vi "Match-Value Image (Colour).vi"(8 "error in (no error)":errorcluster, 9 "Value":u32(colorbox), 10 "Match":T1, 11 "ARGB Image Source":T2) -> (0 "error out":errorcluster, 3 "Match Destination (duplicate)":T1)   [LabVIEW 2020, in "g_ar_toolkit.image.lvlib"]
uses:
  g_ar_toolkit.image.lvlib
  ARGB Image.ctl
  Greyscale Image.ctl
  5701baee-35e2-4306-9a77-a9fdbb5b3a7f.vi
  g_ar_toolkit.common/Module Path.vi
  <vilib>/Utility/error.llb/Error Cluster From Error Code.vi
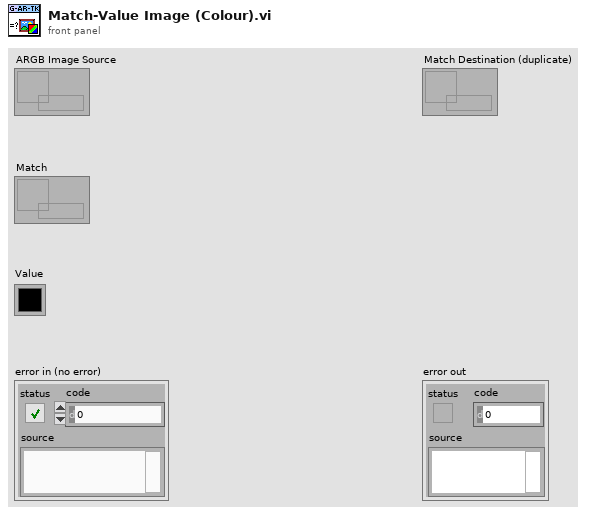
[diagram p1: front panel]
types:
  T1 = typedef "g_ar_toolkit.image.lvlib/Greyscale Image.ctl" = refnum<data-value>
  T2 = typedef "g_ar_toolkit.image.lvlib/ARGB Image.ctl" = refnum<data-value>
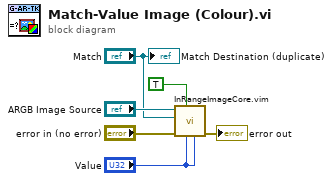
[diagram p0: block diagram]
diagram:
  n1 = call "InRangeImageCore.vim"("Upper"="Value", "Lower"="Value", "IgnoreAlpha"=TRUE, "error in (no error)"="error in (no error)", "In-Range-Result"="Match", "Src"="ARGB Image Source") -> ("error out"=→"error out":errorcluster)  [unwired: 5 in]
  "Match Destination (duplicate)" <- "Match"
